vi "Take and Save Image.vi"(11 "LED Board Visual Test in":refnum<class "LED Board Test.lvclass">) -> (0 "error out":errorcluster, 2 "Color Artifacts Found":bool, 3 "LEDs Found":u32)   [LabVIEW 2015, in "LED Board Test.lvclass"]
uses:
  LED Board Test.lvclass
  CBTF Applications/LED Board Testing/Main/Application/Application/Class/typedefs/Instrument Selector -- Enum.ctl
  Classes/Instruments/Camera/Camera/Class/Camera.lvclass
  LED Board Test.lvclass/LED Board Test.ctl
  Test Class/Test Class.lvclass
  Classes/Application/Class/Application.lvclass
  <vilib>/Cree, Inc/Cree Test Framework/Utilities/Utilities.lvlib
  CBTF Applications/LED Board Testing/Main/Application/Application/Class/LED Board.lvclass
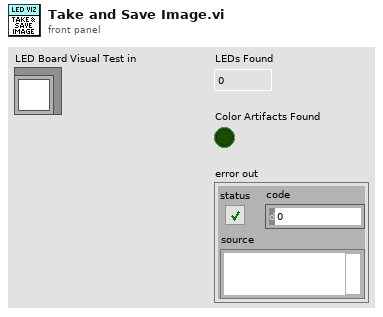
[diagram p1: front panel]
types:
  T1 = typedef "LED Board.lvlib/LED Board.lvclass/Instrument Selector -- Enum.ctl" = enum16{"DC Power Supply 1", "DC Power Supply 2", "DC Power Supply 3", "Camera", "Switch Executive"}
  T2 = typedef "Application.lvlib/App Properties.lvclass/Class Properties -- Cluster.ctl" = cluster{"UUT Info":T3[], "Test Information":refnum<vi>, "Test Complete Event":refnum<user-event>, "Shop Floor System":refnum<class "Shop Floor System.lvclass">, "Gold Board":refnum<class "Golden Board.lvclass">, "Test Recipe":refnum<class "Test Recipe.lvclass">, "Instruments":refnum<class "Instrument.lvclass">[], "Mode":T4, "Test Results":T5[], "Station Config":refnum<class "Station Config.lvclass">}
  T3 = typedef "Application.lvlib/App Properties.lvclass/UUT Reference -- Cluster.ctl" = cluster{"Serial Number Reference":refnum<vi>, "Status Message Reference":refnum<vi>}
  T4 = typedef "Application.lvlib/Application.lvclass/Op Mode -- Enum.ctl" = u16
  T5 = typedef "Application.lvlib/App Properties.lvclass/Test Result -- Cluster.ctl" = cluster{"Position":i32, "Pass":bool, "Fail Codes":string}
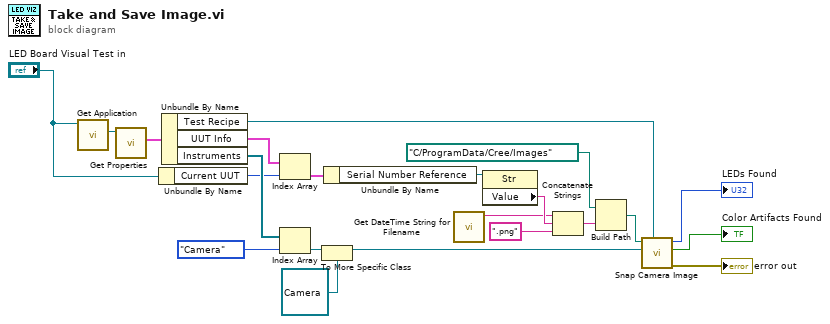
[diagram p0: block diagram]
diagram:
  n1 = call "Get Application.vi"("Test Class in"="LED Board Visual Test in") -> ("Application.lvlib:Application.lvclass"=w18:refnum<class "Application.lvclass">)  [unwired: 9 in, 1 out]
  n2 = call "Get Properties.vi"("Acrobat Template in"=w18) -> ("Class Properties"=w19:T2)  [unwired: 8 in, 2 out]
  n3 = Unbundle By Name("LED Board Visual Test in") -> ("Current UUT"=w6:u32)
  n4 = Unbundle By Name(w19) -> ("Test Recipe"=w1:refnum<class "Test Recipe.lvclass">, "UUT Info"=w16:T3[], "Instruments"=w10:refnum<class "Instrument.lvclass">[])
  n5 = Index Array(array=w16, index=w6) -> (element=w15:T3)
  n6 = Index Array(array=w10, index=Instrument_Selector_--_Enum."Camera" ("Instrument")) -> (element=w8:refnum<class "Instrument.lvclass">)
  n7 = To More Specific Class(target class=refnum<class "Camera.lvclass"> refnum ("Camera.lvlib:Camera.lvclass"), reference=w8) -> (specific class reference=w5:refnum<class "Camera.lvclass">)  [unwired: 1 in, 1 out]
  n8 = Unbundle By Name(w15) -> ("Serial Number Reference"=w14:refnum<vi>)
  n9 = call <vilib>:"Get DateTime String for Filename.vi"() -> ("Date Time String"=w11:string)  [unwired: 11 in]
  n10 = property class="Str"(reference=w14) -> ("Value"=w13:string)  [unwired: 1 in, 2 out]
  n11 = Concatenate Strings(w11, w13, ".png" ("format string")) -> (w22:string)
  n12 = Build Path(base path=path "C:/ProgramData/Cree/Images", name or relative path=w22) -> (appended path=w21:path)
  n13 = call "Snap Camera Image.vi"("Test Recipe in"=w1, "Camera"=w5, "Path"=w21) -> ("error out"=→"error out":errorcluster, "Color Artifacts Found"=→"Color Artifacts Found":bool, "LEDs Found"=→"LEDs Found":u32)  [unwired: 6 in]
